vi "Select Trigger.vi"(8 "Stop Trigger Terminal":T1, 9 "Advance Trigger Terminal":T1, 10 "Period Trigger Terminal":T1, 11 "Acquisition Trigger Terminal":T1) -> (3 "Trigger Signals":T2)   [LabVIEW 2014]
uses:
  Trigger Input Terminals.ctl
  Trigger Signals.ctl
  <vilib>/rvi/eio/common/nirviEmuTemplateMethod_errors.vi
  <vilib>/eio/EIONode/EIONode.xnode
panel:
  # "Copyright 2014 Vidrio Technologies\nScanImage 5 software is licensed under the Apache License, Version 2.0 (the \"License\"); you may not use any files contained\nwithin the ScanImage 5 release except in compliance with the License. You may obtain a copy of the License at\n http://www.apache.org/licenses/LICENSE-2.0\nUnless required by applicable law or agreed to in writing, software distributed under the License is distributed on an\n\"AS IS\" BASIS, WITHOUT WARRANTIES OR CONDITIONS OF ANY KIND, either express or implied. See the License for the\n specific language governing permissions and limitations under the License."
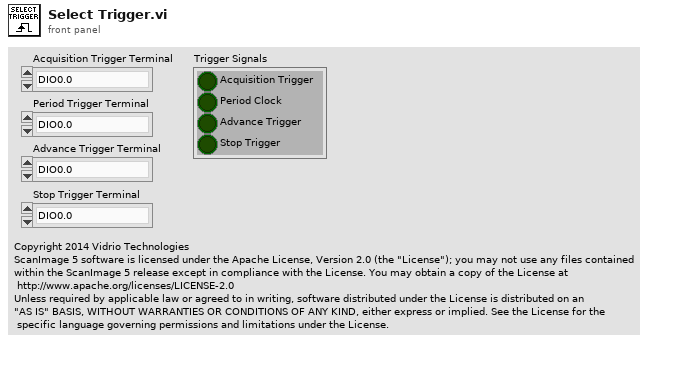
[diagram p1: front panel]
types:
  T1 = typedef "Trigger Input Terminals.ctl" = enum8{"DIO0.0", "DIO0.1", "DIO0.2", "DIO0.3", "PXI_Trig0", "PXI_Trig1", "PXI_Trig2", "PXI_Trig3", "PXI_Trig4", "PXI_Trig5", "PXI_Trig6", "PXI_Trig7", ""}
  T2 = typedef "Trigger Signals.ctl" = cluster{"Acquisition Trigger":bool, "Period Clock":bool, "Advance Trigger":bool, "Stop Trigger":bool}
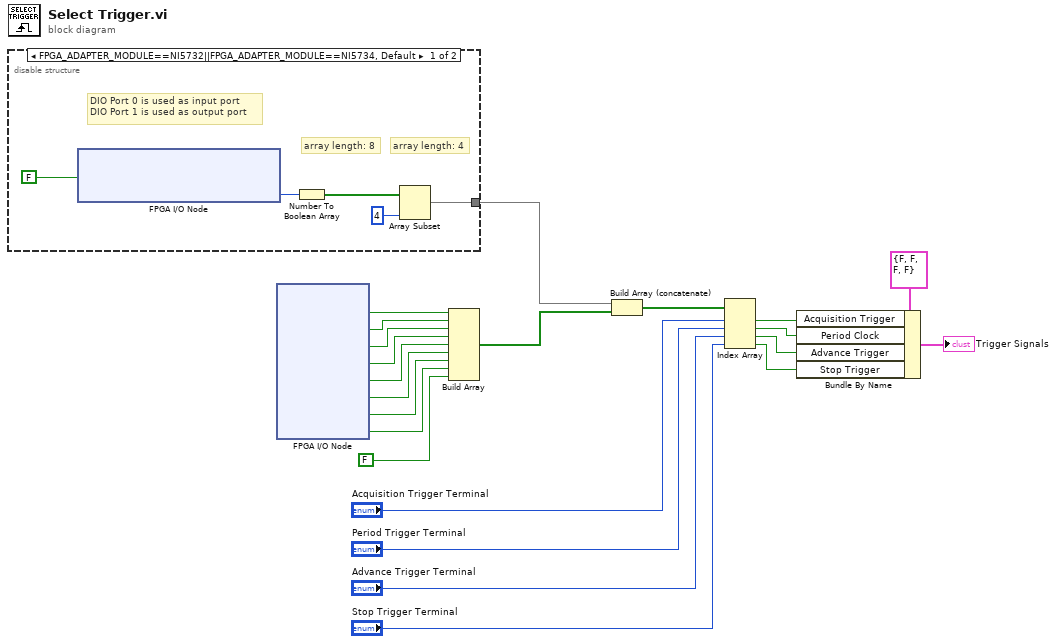
[diagram p0: block diagram]
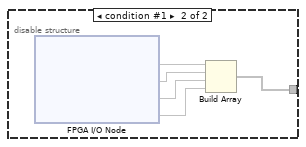
[diagram p2: hidden frame]
diagram:
  n1 = disable-structure shown="FPGA_ADAPTER_MODULE==NI5732||FPGA_ADAPTER_MODULE==NI5734, Default" {
    disable-tunnel: [w23 w28] -> w3
    frame condition #0 (active) {
      # "array length: 4"
      # "array length: 8"
      # "DIO Port 0 is used as input port\nDIO Port 1 is used as output port"
      n2 = xnode "FPGA I/O Node"("IO Module\\DIO Port 0 WE"=FALSE ("IO Module\\DIO Port 0 WE")) -> ("IO Module\\DIO Port 0 Rd Data"=w26:u8)  [unwired: 2 in, 2 out]
      n3 = Number To Boolean Array(number=w26) -> (Boolean array=w24:bool[])
      n4 = Array Subset(array=w24, length=4) -> (w23:bool[])  [unwired: 1 in]
    }
    frame condition #1 {
      n5 = xnode "FPGA I/O Node"() -> ("IO Module\\DI 0"=w32, "IO Module\\DI 1"=w31, "IO Module\\DI 2"=w30, "IO Module\\DI 3"=w29)  [unwired: 4 in, 4 out]
      n6 = Build Array(w32, w31, w30, w29) -> (w28:void[])
    }
  }
  n7 = xnode "FPGA I/O Node"() -> ("PXI_Trig0"=w15:bool, "PXI_Trig1"=w16:bool, "PXI_Trig2"=w17:bool, "PXI_Trig3"=w22:bool, "PXI_Trig4"=w18:bool, "PXI_Trig5"=w19:bool, "PXI_Trig6"=w20:bool, "PXI_Trig7"=w21:bool)  [unwired: 8 in, 8 out]
  n8 = Build Array(w15, w16, w17, w22, w18, w19, w20, w21, FALSE ("element")) -> (w2:bool[])
  n9 = Build Array (concatenate)(w3, w2) -> (w1:bool[])
  n10 = Index Array(array=w1, index #1="Acquisition Trigger Terminal", index #2="Period Trigger Terminal", index #3="Advance Trigger Terminal", index #4="Stop Trigger Terminal") -> (element #1=w11:bool, element #2=w10:bool, element #3=w5:bool, element #4=w4:bool)
  n11 = Bundle By Name(cluster=T2 {"Acquisition Trigger"=FALSE, "Period Clock"=FALSE, "Advance Trigger"=FALSE, "Stop Trigger"=FALSE} ("Trigger"), "Acquisition Trigger"=w11, "Period Clock"=w10, "Advance Trigger"=w5, "Stop Trigger"=w4) -> (→"Trigger Signals":T2)
